vi "FRCts20_Backend_INI_Write_Debug.vi"(8 "error in (no error)":errorcluster, 9 "Save? (T)":bool=TRUE, 10 "debug? (F)":bool, 11 "INI Controller in":refnum<class "FRCts20_Backend_INI Controller.lvclass">) -> (0 "error out":errorcluster, 3 "INI Controller out":refnum<class "FRCts20_Backend_INI Controller.lvclass">)   [LabVIEW 2014, in "FRCts20_Backend_Engine.lvlib" / "FRCts20_Backend_INI Controller.lvclass"]
uses:
  FRCts20_Backend_INI Controller.lvclass
  FRCts20_Backend_INI Controller.lvclass/FRCts20_Backend_INI Controller.ctl
  <vilib>/Utility/config.llb/Write Key (Boolean).vi
  <vilib>/Utility/config.llb/NI_LVConfig.lvlib
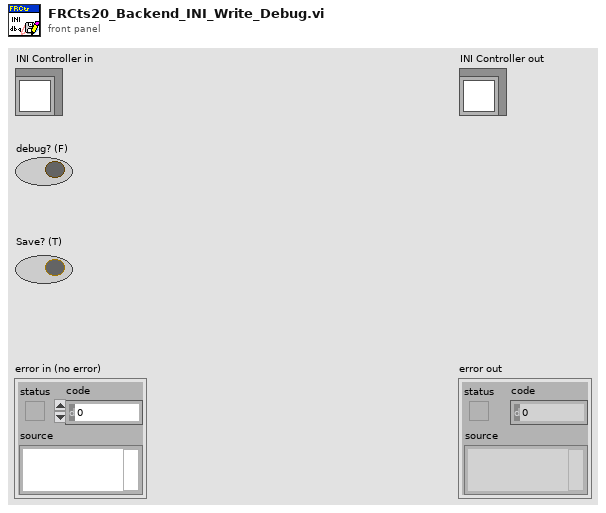
[diagram p1: front panel]
types:
  T1 = typedef "NI_LVConfig.lvlib/Config Data RefNum.ctl" = refnum<k1>
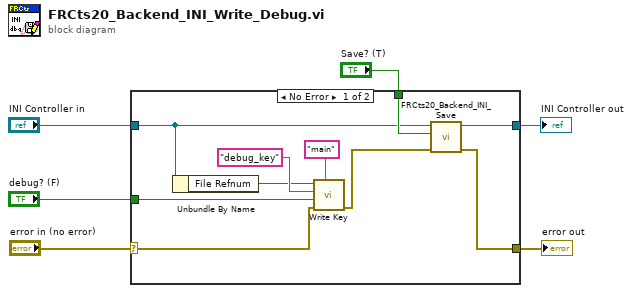
[diagram p0: block diagram]
diagram:
  n1 = case shown="No Error" "error in (no error)" {
    selector: "error in (no error)" -> [w8 w17]
    tunnel: [w14 w17] -> w5
    tunnel: [w16 w18] -> w3
    tunnel: "INI Controller in" -> [w13 w18]
    tunnel: "debug? (F)" -> [w9 _]
    tunnel: "Save? (T)" -> [w15 _]
    frame No Error {
      n2 = Unbundle By Name(w13) -> ("File Refnum"=w10:T1)
      n3 = call-poly <vilib>:"Write Key.vi"("section"="main", "error in (no error)"=w8, "value"=w9, "key"="debug_key", "refnum"=w10) -> ("error out"=w7:errorcluster)  [unwired: 4 in, 2 out]
      n4 = call "FRCts20_Backend_INI_Save.vi"("error in (no error)"=w7, "Save? (T)"=w15, "INI Controller in"=w13) -> ("error out"=w14:errorcluster, "INI Controller out"=w16:refnum<class "FRCts20_Backend_INI Controller.lvclass">)  [unwired: 7 in]
    }
    frame Error {
    }
  }
  "error out" <- w5
  "INI Controller out" <- w3
